vi "App.OpenWaveformDefinition.vi"(7 "StationID":string, 8 "error in (no error)":errorcluster, 11 "selected path":path) -> (0 "error out":errorcluster, 3 "Settings":T1)   [LabVIEW 2015, in "Single Station Execution.lvlib"]
uses:
  Single Station Execution.lvlib
  Types/Saved.Sequence.ctl
  Types/Channel.Properties.ctl
  NationalInstruments.VeriStand
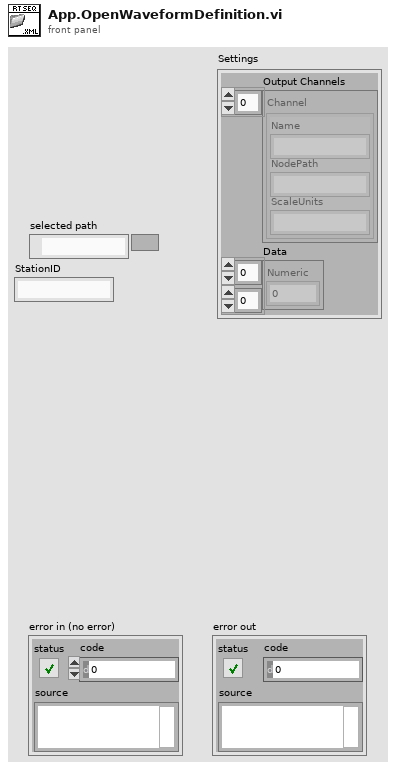
[diagram p1: front panel]
types:
  T1 = typedef "Single Station Execution.lvlib/Saved.Sequence.ctl" = cluster{"Output Channels":T2[], "Data":dbl[][]}
  T2 = typedef "Single Station Execution.lvlib/Channel.Properties.ctl" = cluster{"Name":string, "NodePath":string, "ScaleUnits":string}
  T3 = enum16{"open", "replace", "create", "open or create", "replace or create", "replace or create with confirmation"}
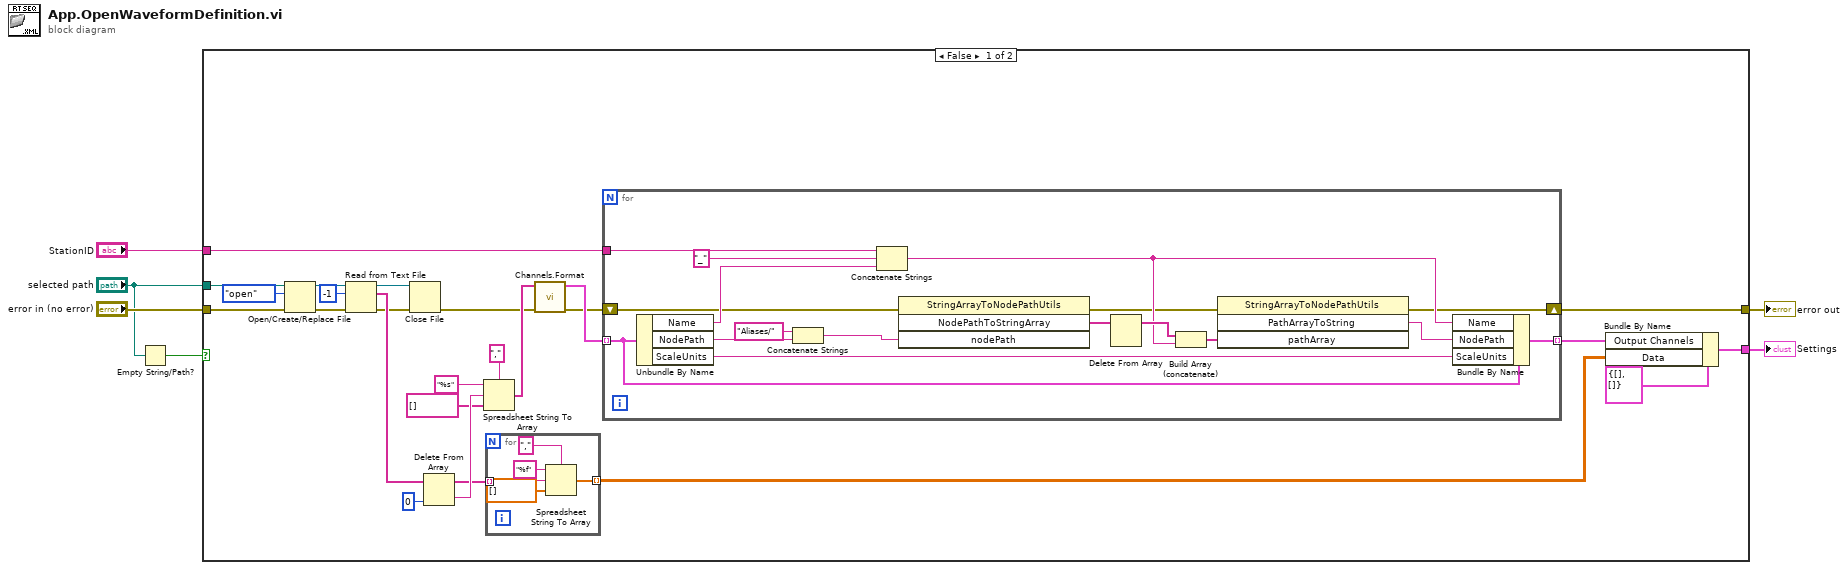
[diagram p0: block diagram]
diagram:
  n1 = Empty String/Path?(string/path="selected path") -> (empty?=w2:bool)
  n2 = case shown="False" w2 {
    tunnel: "error in (no error)" -> [w31 w54]
    tunnel: [w17 _] -> w5
    tunnel: [w7 w54] -> w4
    tunnel: "selected path" -> [w12 _]
    tunnel: "StationID" -> [w9 _]
    frame False {
      n3 = Open/Create/Replace File(file path (use dialog)=w12, error in=w31, operation (0:open)=T3."open") -> (refnum out=w29:refnum<file>, error out=w28:errorcluster)  [unwired: 3 in, 1 out]
      n4 = Read from Text File(file (use dialog)=w29, count=-1, error in=w28) -> (refnum out=w13:refnum<file>, text=w26:string[], error out=w15:errorcluster)  [unwired: 1 in, 1 out]
      n5 = Close File(refnum=w13, error in=w15) -> (error out=w14:errorcluster)  [unwired: 1 out]
      n6 = Delete From Array(array=w26, index=0) -> (deleted portion=w24:string, array with subset deleted=w20:string[])  [unwired: 1 in]
      n7 = Spreadsheet String To Array(delimiter (Tab)=",", format string="%s", spreadsheet string=w24, array type (2D Dbl)=string[] []) -> (array=w18:string[])
      n8 = for {
        tunnel: w20 -> [w53] mode=indexing
        tunnel: [w49] -> w16 mode=indexing
        n9 = Spreadsheet String To Array(delimiter (Tab)=",", format string="%f", spreadsheet string=w53, array type (2D Dbl)=dbl[] []) -> (array=w49:dbl[])
      }
      n10 = call "Channels.Format.vi"("error in (no error)"=w14, "Channels"=w18) -> ("error out"=w8:errorcluster, "Channels (no blanks)"=w11:T2[])  [unwired: 7 in, 1 out]
      n11 = for {
        tunnel: w11 -> [w47] mode=indexing
        tunnel: w9 -> [w44]
        tunnel: [w45] -> w10 mode=indexing
        shift-right: [w34] -> w7
        shift-left: w8 -> [w35]
        n12 = Unbundle By Name(w47) -> ("Name"=w48:string, "NodePath"=w41:string, "ScaleUnits"=w46:string)
        n13 = Concatenate Strings("Aliases/" ("string"), w41) -> (w33:string)
        n14 = Concatenate Strings(w44, "_" ("string"), w48) -> (w39:string)
        n15 = invoke class="StringArrayToNodePathUtils" method="NodePathToStringArray"(error in=w35, "nodePath"=w33) -> (error out=w36:errorcluster, "NodePathToStringArray"=w42:string[])  [unwired: 2 in, 2 out]
        n16 = Delete From Array(array=w42) -> (array with subset deleted=w40:string[])  [unwired: 2 in, 1 out]
        n17 = Build Array (concatenate)(w40, w39) -> (w38:string[])
        n18 = invoke class="StringArrayToNodePathUtils" method="PathArrayToString"(error in=w36, "pathArray"=w38) -> (error out=w34:errorcluster, "PathArrayToString"=w37:string)  [unwired: 2 in, 2 out]
        n19 = Bundle By Name(cluster=w47, "Name"=w39, "NodePath"=w37, "ScaleUnits"=w46) -> (w45:T2)
      }
      n20 = Bundle By Name(cluster=T1 {"Output Channels"=[], "Data"=[]} ("Settings"), "Output Channels"=w10, "Data"=w16) -> (w17:T1)
    }
    frame True {
    }
  }
  "error out" <- w4
  "Settings" <- w5
